vi "Core.vi"(10 "Transaction LUT":refnum<data-value>, 11 "CMD Queue":refnum<queue>) -> ()   [LabVIEW 2012, in "MB Master.lvlib" / "MB_Master_TCP.lvclass"]
uses:
  MB_Master_TCP.lvclass
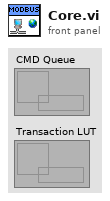
[diagram p1: front panel]
types:
  T1 = cluster{"Data":string, "Notifier":refnum<notifier>}
  T2 = cluster{"IP Address":string, "Port":u16, "Timeout":i32, "Notifier":refnum<notifier>}
  T3 = enum16{"Standard", "Buffered", "CRLF", "Immediate"}
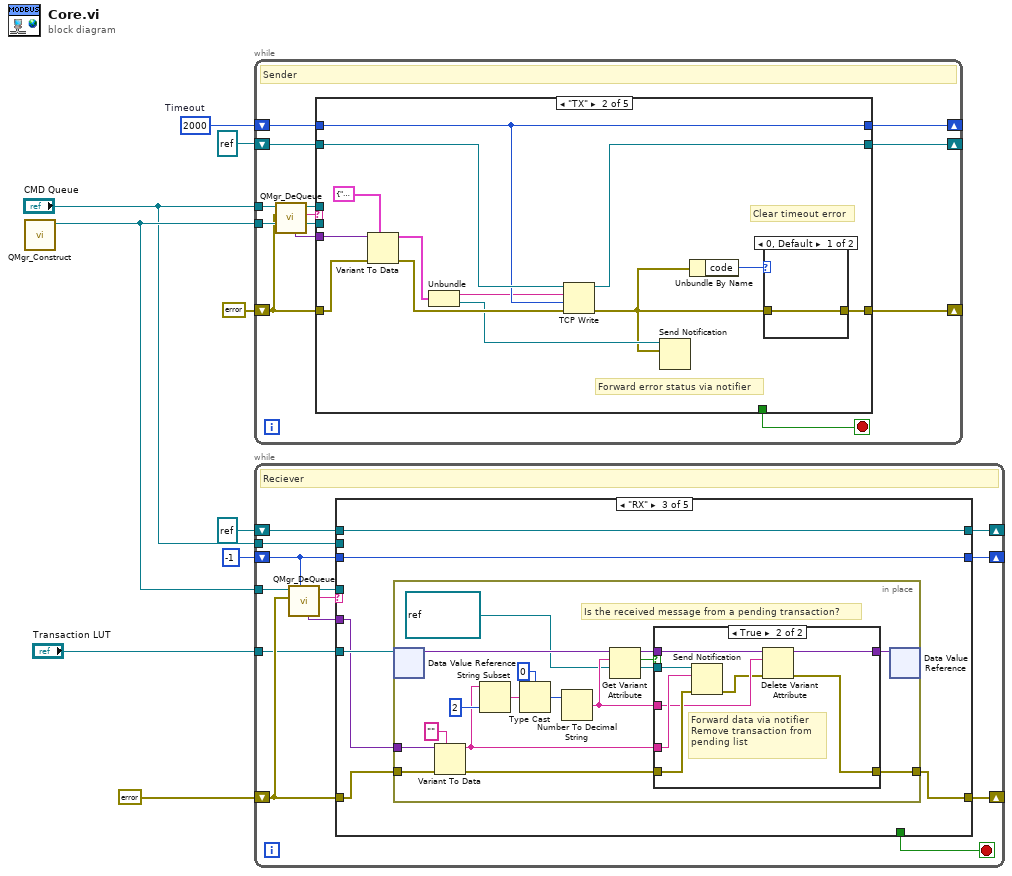
[diagram p0: block diagram]
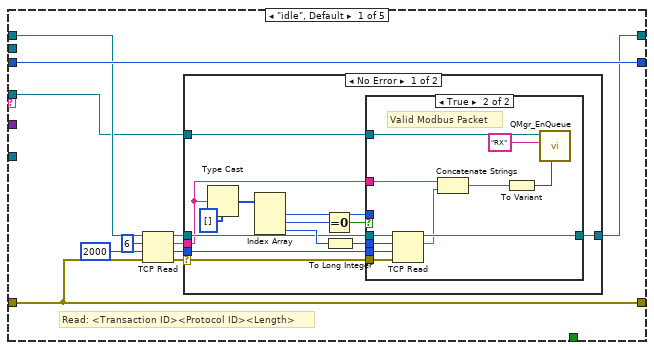
[diagram p2: hidden frame]
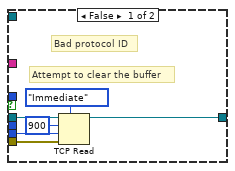
[diagram p3: hidden frame]
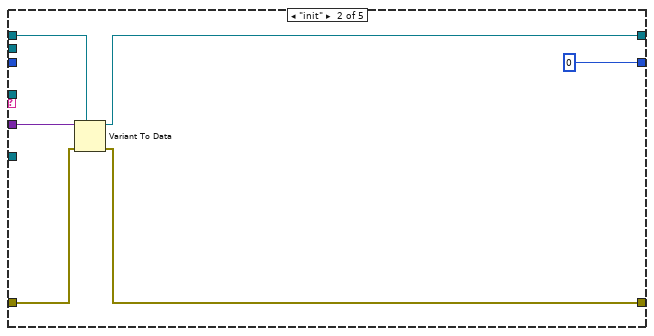
[diagram p5: hidden frame]
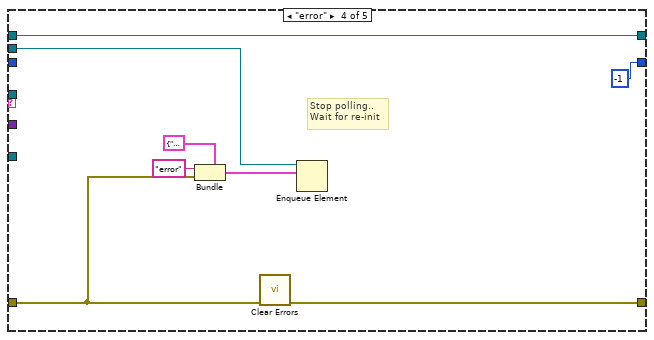
[diagram p7: hidden frame]
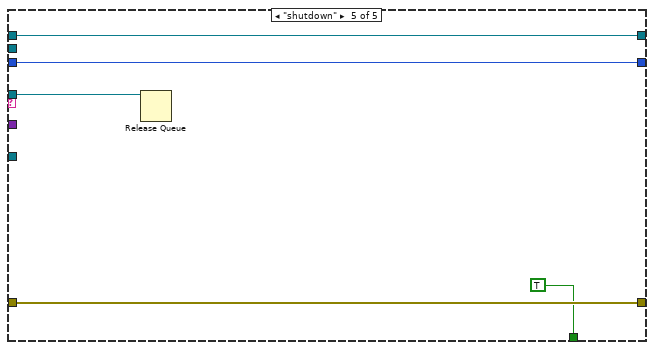
[diagram p8: hidden frame]
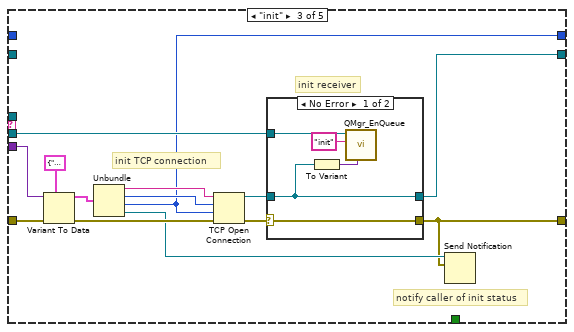
[diagram p11: hidden frame]
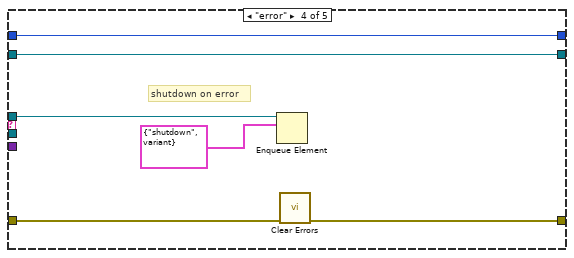
[diagram p13: hidden frame]
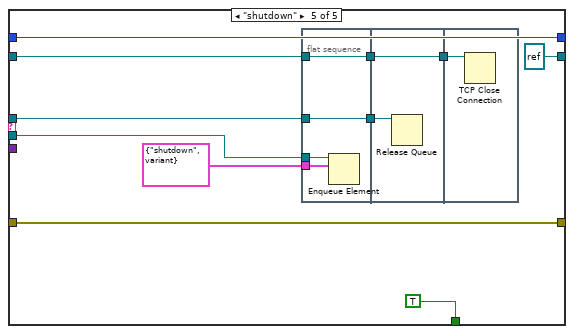
[diagram p14: hidden frame]
diagram:
  w2 = 2000  # Timeout
  n1 = call "QMgr_Construct.vi"() -> ("queue out"=w8:refnum<queue>)  [unwired: 11 in]
  n2 = while {
    tunnel: w8 -> [w21]
    tunnel: "CMD Queue" -> [w20]
    shift-right: [w13] -> _
    shift-left: errorcluster {"status"=FALSE, "code"=0, "source"=""} ("error IO") -> [w14]
    shift-right: [w16] -> _
    shift-left: refnum<k5> refnum ("TCP connection in") -> [w15]
    shift-right: [w11] -> _
    shift-left: w2 -> [w10]
    stop <- w12 stop-if-true
    # "Sender"
    n3 = call "QMgr_DeQueue.vi"("error in (no error)"=w14, "queue in"=w20) -> ("Command"=w19:string, "queue out"=w18:refnum<queue>, "data"=w17:variant)  [unwired: 7 in]
    n4 = case shown="\"TX\"" w19 {
      tunnel: w21 -> [_ _ w52 _ w69]
      tunnel: w18 -> [_ _ _ w64 w71]
      tunnel: w17 -> [_ w37 w46 _ _]
      tunnel: w14 -> [w23 w36 w48 w62 w67]
      tunnel: [w24 w33 w49 w65 refnum<k5> refnum ("TCP connection in")] -> w16
      tunnel: w15 -> [w24 w35 _ w65 w74]
      tunnel: [w23 w25 w40 w61 w67] -> w13
      tunnel: [_ _ _ _ TRUE] -> w12
      tunnel: [w22 w32 w39 w60 w66] -> w11
      tunnel: w10 -> [w22 w32 _ w60 w66]
      frame "idle", Default {
      }
      frame "TX" {
        # "Forward error status via notifier"
        # "Clear timeout error"
        n5 = Variant To Data(error in=w36, type=T1 {"Data"="", "Notifier"=refnum}, Variant=w37) -> (data=w30:T1, error out=w34:errorcluster)
        n6 = Unbundle(w30) -> ("Data"=w29:string, "Notifier"=w28:refnum<notifier>)
        n7 = TCP Write(connection ID=w35, data in=w29, error in (no error)=w34, 9:w32) -> (connection ID out=w33:refnum<k5>, error out=w26:errorcluster)  [unwired: 1 out]
        n8 = Send Notification(notification=w26, notifier=w28) -> ()  [unwired: 1 in, 2 out]
        n9 = Unbundle By Name(w26) -> ("code"=w27:i32)
        n10 = case shown="0, Default" w27 {
          tunnel: w26 -> [w38 _]
          tunnel: [w38 _] -> w25
          frame 0, Default {
          }
          frame 56 {
          }
        }
      }
      frame "init" {
        # "notify caller of init status"
        # "init receiver"
        # "init TCP connection"
        n11 = Variant To Data(error in=w48, type=T2 {"IP Address"="", "Port"=502, "Timeout"=10000, "Notifier"=refnum}, Variant=w46) -> (data=w45:T2, error out=w42:errorcluster)
        n12 = Unbundle(w45) -> ("IP Address"=w44:string, "Port"=w43:u16, "Timeout"=w39:i32, "Notifier"=w41:refnum<notifier>)
        n13 = TCP Open Connection(address=w44, remote port or service name=w43, timeout ms (60000)=w39, error in (no error)=w42) -> (connection ID=w51:refnum<k5>, error out=w50:errorcluster)  [unwired: 1 in]
        n14 = case shown="No Error" w50 {
          selector: w50 -> [w54 w59]
          tunnel: w52 -> [w57 _]
          tunnel: w51 -> [w53 w58]
          tunnel: [w54 w59] -> w40
          tunnel: [w53 w58] -> w49
          frame No Error {
            n15 = To Variant(anything=w53) -> (Variant=w55:variant)
            n16 = call "QMgr_EnQueue.vi"("Data"=w55, "Command"="init", "queue in"=w57) -> ()  [unwired: 8 in, 1 out]
          }
          frame Error {
          }
        }
        n17 = Send Notification(notification=w40, notifier=w41) -> ()  [unwired: 1 in, 2 out]
      }
      frame "error" {
        # "shutdown on error"
        n18 = Enqueue Element(queue=w64, element=cluster{"cmd":string, "data":variant} {"cmd"="shutdown", "data"=variant}) -> ()  [unwired: 2 in, 3 out]
        n19 = call <vilib>:"Clear Errors.vi"("error in (no error)"=w62) -> ("error out"=w61:errorcluster)  [unwired: 6 in]
      }
      frame "shutdown" {
        n20 = flat-sequence {
          tunnel: w74 -> [w80]
          tunnel: [w80] -> w73
          tunnel: w71 -> [w79]
          tunnel: [w79] -> w70
          tunnel: w69 -> [w78]
          tunnel: cluster{"cmd":string, "data":variant} {"cmd"="shutdown", "data"=variant} ("element") -> [w77]
          tunnel: w73 -> [w82]
          tunnel: [w82] -> w72
          tunnel: w70 -> [w81]
          tunnel: w72 -> [w83]
          frame #0 {
            n21 = Enqueue Element(queue=w78, element=w77) -> ()  [unwired: 2 in, 3 out]
          }
          frame #1 {
            n22 = Release Queue(queue=w81) -> ()  [unwired: 2 in, 3 out]
          }
          frame #2 {
            n23 = TCP Close Connection(connection ID=w83) -> ()  [unwired: 2 in, 2 out]
          }
        }
      }
    }
  }
  n24 = while {
    tunnel: w8 -> [w96]
    shift-right: [w95] -> _
    shift-left: errorcluster {"status"=FALSE, "code"=0, "source"=""} ("error in (no error)") -> [w94]
    shift-right: [w88] -> _
    shift-left: -1 ("timeout in ms (-1)") -> [w89]
    shift-right: [w86] -> _
    shift-left: refnum<k5> refnum ("TCP connection in") -> [w87]
    tunnel: "CMD Queue" -> [w85]
    tunnel: "Transaction LUT" -> [w84]
    stop <- w90 stop-if-true
    # "Reciever"
    n25 = call "QMgr_DeQueue.vi"("timeout in ms (-1)"=w89, "error in (no error)"=w94, "queue in"=w96) -> ("Command"=w93:string, "queue out"=w91:refnum<queue>, "data"=w92:variant)  [unwired: 6 in]
    n26 = case shown="\"RX\"" w93 {
      tunnel: w94 -> [w100 w143 w148 w179 w189]
      tunnel: [w100 w142 w145 w184 w189] -> w95
      tunnel: w92 -> [_ w141 w144 _ _]
      tunnel: w91 -> [w97 _ _ _ w187]
      tunnel: [_ _ _ _ TRUE] -> w90
      tunnel: w89 -> [w106 _ w146 _ w185]
      tunnel: [w106 0 ("timeout in ms (-1)") w146 -1 ("timeout in ms (-1)") w185] -> w88
      tunnel: w87 -> [w105 w140 w147 w183 w186]
      tunnel: [w101 w139 w147 w183 w186] -> w86
      tunnel: w85 -> [_ _ _ w177 _]
      tunnel: w84 -> [_ _ w149 _ _]
      frame "idle", Default {
        w103 = 2000 ("timeout ms (25000)")
        # "Read: <Transaction ID><Protocol ID><Length>"
        n27 = TCP Read(connection ID=w105, bytes to read=6, error in (no error)=w100, 9:w103) -> (connection ID out=w102:refnum<k5>, data out=w99:string, error out=w98:errorcluster)  [unwired: 1 in]
        n28 = case shown="No Error" w98 {
          selector: w98 -> [w108 _]
          tunnel: w103 -> [w115 _]
          tunnel: w102 -> [w113 w137]
          tunnel: [w111 w137] -> w101
          tunnel: w99 -> [w109 _]
          tunnel: w97 -> [w107 _]
          frame No Error {
            n29 = Type Cast(type=u16[] [], x=w109) -> (*(type *) &x=w118:u16[])
            n30 = Index Array(array=w118) -> (element #1=w110:u16, element #2=w116:u16, element #3=w119:u16)  [unwired: 3 in]
            n31 = Equal To 0?(x=w116) -> (x = 0?=w112:bool)
            n32 = To Long Integer(number=w119) -> (32bit integer=w114:i32)
            n33 = case shown="True" w112 {
              tunnel: w108 -> [w121 w136]
              tunnel: w115 -> [w124 w135]
              tunnel: w114 -> [_ w134]
              tunnel: w113 -> [w125 w133]
              tunnel: [w122 w132] -> w111
              tunnel: w107 -> [_ w131]
              tunnel: w110 -> [_ _]
              tunnel: w109 -> [_ w128]
              frame False {
                # "Attempt to clear the buffer"
                # "Bad protocol ID"
                n34 = TCP Read(connection ID=w125, bytes to read=900, error in (no error)=w121, 7:T3."Immediate" ("mode (standard)"), 9:w124) -> (connection ID out=w122:refnum<k5>)  [unwired: 2 out]
              }
              frame True {
                # "Valid Modbus Packet"
                n35 = TCP Read(connection ID=w133, bytes to read=w134, error in (no error)=w136, 9:w135) -> (connection ID out=w132:refnum<k5>, data out=w127:string)  [unwired: 1 in, 1 out]
                n36 = Concatenate Strings(w128, w127) -> (w126:string)
                n37 = To Variant(anything=w126) -> (Variant=w130:variant)
                n38 = call "QMgr_EnQueue.vi"("Data"=w130, "Command"="RX", "queue in"=w131) -> ()  [unwired: 8 in, 1 out]
              }
            }
          }
          frame Error {
          }
        }
      }
      frame "init" {
        n39 = Variant To Data(error in=w143, type=w140, Variant=w141) -> (data=w139:refnum<k5>, error out=w142:errorcluster)
      }
      frame "RX" {
        n40 = in-place {
          in-place-border: w144 -> [w166]
          in-place-border: w148 -> [w165]
          in-place-border: [w153] -> w145
          # "Is the received message from a pending transaction?"
          n41 = in-place-dvr #1(w149) -> (w152:variant)  [unwired: 1 out]
          n42 = Variant To Data(error in=w165, type="", Variant=w166) -> (data=w157:string, error out=w156:errorcluster)
          n43 = String Subset(string=w157, length (rest)=2 ("length (rest)")) -> (substring=w162:string)  [unwired: 1 in]
          n44 = Type Cast(type=u16 0, x=w162) -> (*(type *) &x=w160:u16)
          n45 = Number To Decimal String(number=w160) -> (decimal integer string=w154:string)  [unwired: 1 in]
          n46 = Get Variant Attribute(Variant=w152, name=w154, default value (empty Variant)=refnum<notifier> refnum ("notifier")) -> (duplicate Variant=w158:variant, found=w159:bool, value=w155:refnum<notifier>)  [unwired: 1 in, 1 out]
          n47 = case shown="True" w159 {
            tunnel: w158 -> [w168 w173]
            tunnel: w157 -> [_ w175]
            tunnel: w156 -> [w167 w174]
            tunnel: w155 -> [_ w176]
            tunnel: w154 -> [_ w172]
            tunnel: [w167 w170] -> w153
            tunnel: [w168 w169] -> w151
            frame False {
              # "Ignore the message"
            }
            frame True {
              # "Forward data via notifier\nRemove transaction from\npending list"
              n48 = Send Notification(notification=w175, notifier=w176, error in (no error)=w174) -> (error out=w171:errorcluster)  [unwired: 1 out]
              n49 = Delete Variant Attribute(4:w171, 6:w172, 7:w173) -> (0:w170:errorcluster, 3:w169:variant)  [unwired: 1 out]
            }
          }
          n50 = in-place-dvr #1(w151) -> ()  [unwired: 2 out]
        }
      }
      frame "error" {
        # "Stop polling..\nWait for re-init"
        n51 = Bundle(cluster=cluster{"cmd":string, "data":variant} {"cmd"="shutdown", "data"=variant} ("element"), "cmd"="error", "data"=w179) -> (w178:cluster{"cmd":string, "data":variant})
        n52 = call <vilib>:"Clear Errors.vi"("error in (no error)"=w179) -> ("error out"=w184:errorcluster)  [unwired: 6 in]
        n53 = Enqueue Element(queue=w177, element=w178) -> ()  [unwired: 2 in, 3 out]
      }
      frame "shutdown" {
        n54 = Release Queue(queue=w187) -> ()  [unwired: 2 in, 3 out]
      }
    }
  }
